vi "T90 Test Konfig.vi"() -> ()   [LabVIEW 2020, in "EPA 1065.lvlib" / "T90 Test 1065-308.lvlib"]
uses:
  T90 Test 1065-308.lvlib
  T90 Konfig Daten.ctl
  Modus.ctl
  Seiten/System Einstellungen V2/Analysatoren.ctl
  Seiten/System Einstellungen V2/Gasflasche Auswahl.ctl
  Seiten/System Einstellungen V2/Konfig Gasflasche.ctl
  Frequenz.ctl
  Visualisierungs Elemente/Zahlen-Ausgabefeld.ctl
  Ergebnis.ctl
  Aktion FGV T90.ctl
  Seiten/FT-IR/FGV FT-IR Gasliste Aktionen.ctl
  Aktion T90 Zustandsautomat.ctl
  Sprachverwaltung/FGV Aktion Tabelle zerlegen.ctl
  Seiten/System Einstellungen V2/Aktion FGV Gasbottledefinition.ctl
  PDF_Interface/PDF Interface Helper/PDFResultPictures.ctl
  Aktion FGV Datenmanagment.ctl
  Allgemeine VIs/Aktion Wertaenderung Gasliste.ctl
  Result Textfile.ctl
  Allgemeine VIs/Aktion Test Status.ctl
  Funktionstasten/Funktionstasten-Aktion.ctl
  Funktionstasten/Zustaende.ctl
  Allgemein/allgemeine Sub-VIs.lvlib
  Seiten/FT-IR/FT-IR.lvlib
  Funktionstasten/Funktionstasten.lvlib
  Linearisierung V2/Protokoll/Protokoll.lvlib
  EPA 1065.lvlib
  Sprachverwaltung/Sprachverwaltung.lvlib
  Seiten/System Einstellungen V2/System Einstellungen V2.lvlib
  PDF_Interface/PDF Interface Helper/PDF Interface Helper.lvlib
  Seiten/Gaszuordnung AO/Gaszuordnung AO.lvlib
panel:
  out "Ergebnis PDF FALSE":T1 caption="Ergebnis 2"
  out "Ergebnis PDF TRUE":T1 caption="Ergebnis 1"
  out "T90 PDF":waveform(sgl)(graph) caption="T90"
  in  "Systemeinstellung":bool caption="Gasliste geändert"
  in  "Gasliste geändert":bool
  in  "Registerkarte":enum32{"Settings", "T90 Test", "Result"}(tab)
  in  "T90 Konfig Daten":T2={"Bearbeiter:"="", "Komponente:"=0, "Gasflaschen Nr.:"="", "Accuracy"=0.0, "Sollwert"=0.0, "Modus"=0, "Abschaltzeit:"=120.0, "Abweichung:"=3.0, "Pfad:"=path "D:/IAG_Data/Log", "Textname:"="", "CG Aufschaltzeit:"=120.0, "Einheit"="", "N2 Aufschaltzeit:"=120.0, "Analysator"="", "Gasflasche"=0, "Konfig Gasflasche"=FALSE, "Frequency:"=5} {"Frequency:" items=["5 Hz"=5, "10 Hz"=10]; "Gasflasche" items=["----"=10000, "IAG O2"=0, "IAG C2H2"=1, "IAG C2H4"=2, "IAG NH3 200"=3, "IAG NH3 2000"=4, "IAG NH3 3000"=5, "IAG CO 5%"=6, "IAG Propane 2%"=7, "IAG NO 1000"=8, "IAG SO2"=9, "IAG C3H6"=10, "IAG CO2"=11, "IAG CO"=12, "IAG N2O"=13, "IAG N2O 100"=14, "IAG NO2 1000"=15, "IAG NO2 100"=16, "IAG CH4"=17, "IAG Propane"=18, "IAG NO 5000"=19, "Hansi"=20, "IAG MG"=21]; "N2 Aufschaltzeit:" min=30.0; "CG Aufschaltzeit:" min=60.0; "Komponente:" items=["NO (3000) LP 191C", "NO2 (150) LP 191C (1of2)", "NO2 (2000) LP 191C (2of2)", "N2O (300) LP 191C (1of2)", "NH3 (300) LP 191C (1of2)", "NH3 (900,3000) LP 191C (2of2)", "HNCO (400) 191C", "H2O% (30) LP 191C", "Formaldehyde (70,500) LP 191C", "CO2 low% (4) LP 191C (2of2)", "CO2% (20) LP 191C (1of2)", "CO (700) LP 191C (1of3)", "CO% (1) LP 191C (2of3)", "Propylene (1000) LP 191C", "Aromatic HC C7 (500) LP 191C", "Ethylene (1000) LP 191C", "CH4 (250) LP 191C (1of2)", "CH4 (5000) LP 191C (2of2)", "Ethane (1000) LP 191C", "Acetylene (1000) LP 191C", "HNO2 (20) 191C", "MeOH (1000) 191C", "CO% (10) LP 191C (3of3)", "Formic Acid (100) 191C", "SO2 (500) LP 191C", "Acetaldehyde (1000) LP 191C", "COS (100) LP 191C", "1,3 butadiene (100) LP 191C", "Oil as Octane (200) LP 191C", "N2O (1000) LP 191C (2of2)", "Propane (200) LP 191C", "NO2 autorange (2000)", "CO autorange (100000)", "CH4 autorange (5000)", "NH3 autorange (3000)", "NOx autorange (3000)", "HCD (10000)", "NMHCD (10000)", "CO2% autorange (20)", "H2Oppm (300000)", "N2O autorange (1000)", "NMNEHCD (3000)", "Temp. Gascell", "Pressure Gascell", "sBeam@2500", "Temp. HL to FT-IR", "Temp. HL Extern SP1", "Outlet Temp FT-IR", "Temp. Cabinet", "Constant 0", "Constant 50", "Constant 100", "AK DUMMY"]; "Abweichung:" min=2.0; "Abschaltzeit:" min=60.0; "Modus" items=["CG zu PNS", "CG zu Entnahmestelle"]}
  in  "Speichern":bool caption="Save"
  out "Komponente":string caption="Komponente:"
  out "Status":string
  out "T90":waveform(sgl)(graph)
  in  "Test Start":bool
  in  "Abbrechen":bool
  out "Istwert":T8 caption="Istwert:" format="%.2f"
  out "Einheit":string
  out "Averaged T10-T90":string caption="gemittelter T10-T90"
  out "Frequenz 2":string
  out "Averaged T90-T10":string caption="gemittelter T90-T10"
  out "Averaged T90-T10 2":string caption="gemittelter T90-T10"
  out "Averaged T10-T90 2":string caption="gemittelter T10-T90"
  out "Ergebnis 4":T1
  out "Ergebnis 3":T1
  out "Ergebnis 2":T1
  out "Ergebnis 1":T1
  out "Ergebnis x5 (T90 T10)":string caption="Mean T10-T90"
  out "Ergebnis x5 (T10 T90)":string caption="Mean T10-T90"
  out "Frequenz 1":string
  out "Tabelle T0-T90":string[][](table) caption="Tabelle"
  in  "Save to file":bool caption="Abbrechen"
  out "T90 Result":waveform(sgl)(graph) caption="T90"
  in  "Print PDF":bool caption="Abbrechen"
  out "Tabelle":string[][](table)
  # "T90 Test EPA §1065.308"
  # "Editor"
  # "Gas bottle number:"
  # "Übersetzungen:\n\nCG priming Time:\nCG Purge Time:"
  # "Path"
  # "Textname:"
  # "Allgemeine Einstellung"
  # "Protokoll Einstellung"
  # "sec."
  # "sec."
  # "%"
  # "%"
  # "sec."
  # "Grenzen"
  # "Ergebnis"
  # "s"
  # ">5"
  # ">5"
  # "<10s"
  # "<10s"
  # "s"
  # "s"
  # "s"
  # "s"
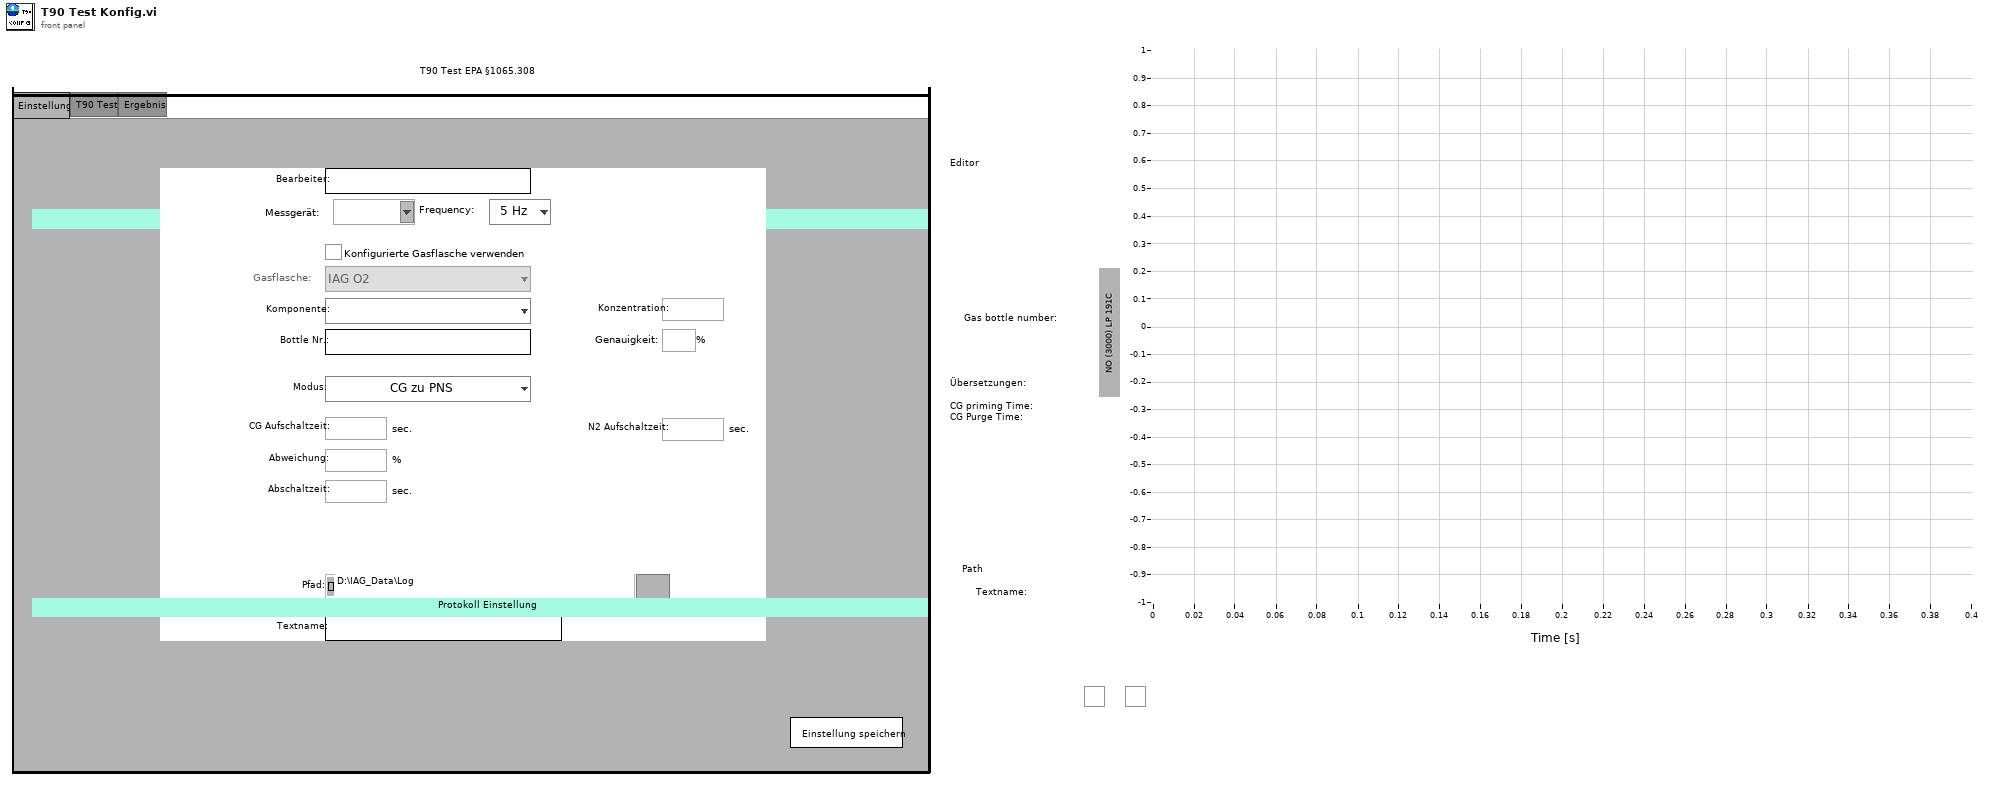
[diagram p1: front panel]
types:
  T1 = typedef "EPA 1065.lvlib/T90 Test 1065-308.lvlib/Ergebnis.ctl" = bool
  T2 = typedef "EPA 1065.lvlib/T90 Test 1065-308.lvlib/T90 Konfig Daten.ctl" = cluster{"Bearbeiter:":string, "Komponente:":u16, "Gasflaschen Nr.:":string, "Accuracy":dbl, "Sollwert":dbl, "Modus":T3, "Abschaltzeit:":dbl, "Abweichung:":dbl, "Pfad:":path, "Textname:":string, "CG Aufschaltzeit:":dbl, "Einheit":string, "N2 Aufschaltzeit:":dbl, "Analysator":T4, "Gasflasche":T5, "Konfig Gasflasche":T6, "Frequency:":T7}
  T3 = typedef "EPA 1065.lvlib/T90 Test 1065-308.lvlib/Modus.ctl" = u16
  T4 = typedef "System Einstellungen V2.lvlib/Analysatoren.ctl" = string
  T5 = typedef "System Einstellungen V2.lvlib/Gasflasche Auswahl.ctl" = u16
  T6 = typedef "System Einstellungen V2.lvlib/Konfig Gasflasche.ctl" = bool
  T7 = typedef "EPA 1065.lvlib/T90 Test 1065-308.lvlib/Frequenz.ctl" = u16
  T8 = typedef "Zahlen-Ausgabefeld.ctl" = sgl
  T9 = typedef "EPA 1065.lvlib/T90 Test 1065-308.lvlib/Aktion FGV T90.ctl" = enum16{"lesen", "Konfig Daten", "speichern", "laden", "T90 aktiv", "T90 inaktiv", "Ext. Ventil aktivieren", "Ext. Ventil deaktivieren", "N2 spülen aktiv", "N2 spülen inaktiv", "Ergebnis Textfile"}
  T10 = typedef "System Einstellungen V2.lvlib/Aktion FGV Gasbottledefinition.ctl" = enum16{"lesen", "schreiben", "löschen", "laden", "speichern", "exportieren", "importieren"}
  T11 = typedef "Sprachverwaltung.lvlib/FGV Aktion Tabelle zerlegen.ctl" = enum16{"laden", "vereinzeln", "speichern"}
  T12 = typedef "EPA 1065.lvlib/T90 Test 1065-308.lvlib/Aktion T90 Zustandsautomat.ctl" = enum16{"init", "start", "CG aufschalten", "Aufschaltzeit einhalten", "Peak ermitteln", "spülen", "CG Sequenz T10", "CG Sequenz T90", "CG halten", "N2 Sequenz T90", "N2 Sequenz T10", "N2 halten", "Auswerten", "abbrechen", "Störung", "fertig"}
  T13 = typedef "FT-IR.lvlib/FGV FT-IR Gasliste Aktionen.ctl" = enum16{"lesen", "Gasliste FT-IR", "Gasliste ausgelesen", "laden", "speichern", "löschen"}
  T14 = typedef "PDF Interface.lvlib/PDF Interface Helper.lvlib/PDFResultPictures.ctl" = cluster{"Yes Ctl Refnum":refnum<vi>, "No Ctl Refnum":refnum<vi>}
  T15 = typedef "String - Ausgabefeld.ctl" = string
  T16 = typedef "System Einstellungen V2.lvlib/Gasflasche gesamt.ctl" = cluster{"Gasflasche":T17, "Trägergas":T18, "Komponenten":T19[]}
  T17 = typedef "System Einstellungen V2.lvlib/Gasflasche.ctl" = cluster{"Gasname für die Auswahl":string, "Chargennummer":string, "Ablaufdatum":timestamp}
  T18 = typedef "System Einstellungen V2.lvlib/Traegergas.ctl" = string
  T19 = typedef "System Einstellungen V2.lvlib/Gasflaschenkomponente.ctl" = cluster{"Gasauswahl":string, "Konzentration IST":dbl, "Einheit":string, "Genauigkeit":dbl}
  T20 = cluster{"Komponente:":u16, "Sollwert":dbl, "Accuracy":dbl, "Einheit":string, "Gasflaschen Nr.:":string}
  T21 = typedef "EPA 1065.lvlib/Aktion Wertaenderung Gasliste.ctl" = enum16{"Init", "lesen", "Gasliste geändert", "ARN inaktiv", "LEAK inaktiv", "Interference 366 inaktiv", "T90 inaktiv", "Interference 375 inaktiv", "Chiller inaktiv", "FID O2 inaktiv", "FID Opti inaktiv", "Drift inaktiv", "Pre Test inaktiv", "LinV2 inaktiv", "HovaCAL Interference inaktiv"}
  T22 = typedef "EPA 1065.lvlib/T90 Test 1065-308.lvlib/Aktion FGV Datenmanagment.ctl" = enum16{"init", "lesen", "Istwerte schreiben", "höchsten Peak setzen", "Auswerten", "Grenzen setzen", "Sollwert ändern", "Rise T10", "Rise T90", "Fall T90", "Fall T10", "Bit löschen", "Umschaltzeitpunkt"}
  T23 = typedef "EPA 1065.lvlib/T90 Test 1065-308.lvlib/Result Textfile.ctl" = cluster{"Averaged T10-T90":string, "Averaged T90-T10":string, "Ergebnis x5 (T10 T90)":string, "Ergebnis x5 (T90 T10)":string, "Ergebnis 1":T1, "Ergebnis 2":T1, "Ergebnis 3":T1, "Ergebnis 4":T1}
  T24 = enum16{"open", "replace", "create", "open or create", "replace or create", "replace or create with confirmation"}
  T25 = typedef "EPA 1065.lvlib/Aktion Test Status.ctl" = enum16{"init", "lesen", "prüfen", "Interference 366", "Interference 375", "Chiller läuft", "Drift läuft", "Pre Test läuft", "FID Optimization läuft", "FID Interference läuft", "HovaCAL Interference", "LinV2"}
  T26 = typedef "Funktionstasten.lvlib/Zustaende.ctl" = enum16{"Standby", "Pause", "Eco", "Messen", "Kalibrieren", "Spülen Filter", "Spülen Leitung", "Umgebungsluft", "0-Gas", "Cal-Gas", "CG zu PNS", "-------------", "Init 1", "Init 2", "Init 3", "Init 4", "Messen vorbereiten", "Messen durchführen", "Exit"}
  T27 = typedef "Funktionstasten.lvlib/Funktionstasten-Aktion.ctl" = enum16{"Initialisieren", "Zustand setzen", "Taste gedrückt", "Fehler speichern", "Lesen", "Manuell", "Remote", "Bitparallel", "Samplepoint", "Zeit Prüfen", "reset Umschalten"}
  T28 = typedef "EPA 1065.lvlib/Aktive Tests Cluster.ctl" = cluster{"ANR läuft":bool, "T90 läuft":bool, "Leak läuft":bool, "Interference 366 läuft":bool, "Interference 375 läuft":bool, "Chiller läuft":bool, "FID Interference läuft":bool, "FID optimization läuft":bool, "Drift läuft":bool, "Pre-test läuft":bool, "HovaCAL Interference läuft":bool, "LinV2 läuft":bool}
  T29 = typedef "EPA 1065.lvlib/T90 Test 1065-308.lvlib/Datencluster.ctl" = cluster{"Höchster Peak":T30, "T10 Grenzwert":T30, "T90 Grenzwert":T30, "Rise Times":dbl[], "Fall Times":dbl[], "RiseTime gemittelt":T30, "FallTime gemittelt":T30, "Zeitstempel":timestamp[], "Rise T10":bool, "Rise T90":bool, "Fall T10":bool, "Fall T90":bool, "RiseTime >5":bool, "Falltime >5":bool, "RiseTime <10":bool, "Falltime <10":bool, "T0-T90":dbl[], "T100-T10":dbl[]}
  T30 = typedef "Zahlen-Eingabefeld.ctl" = sgl
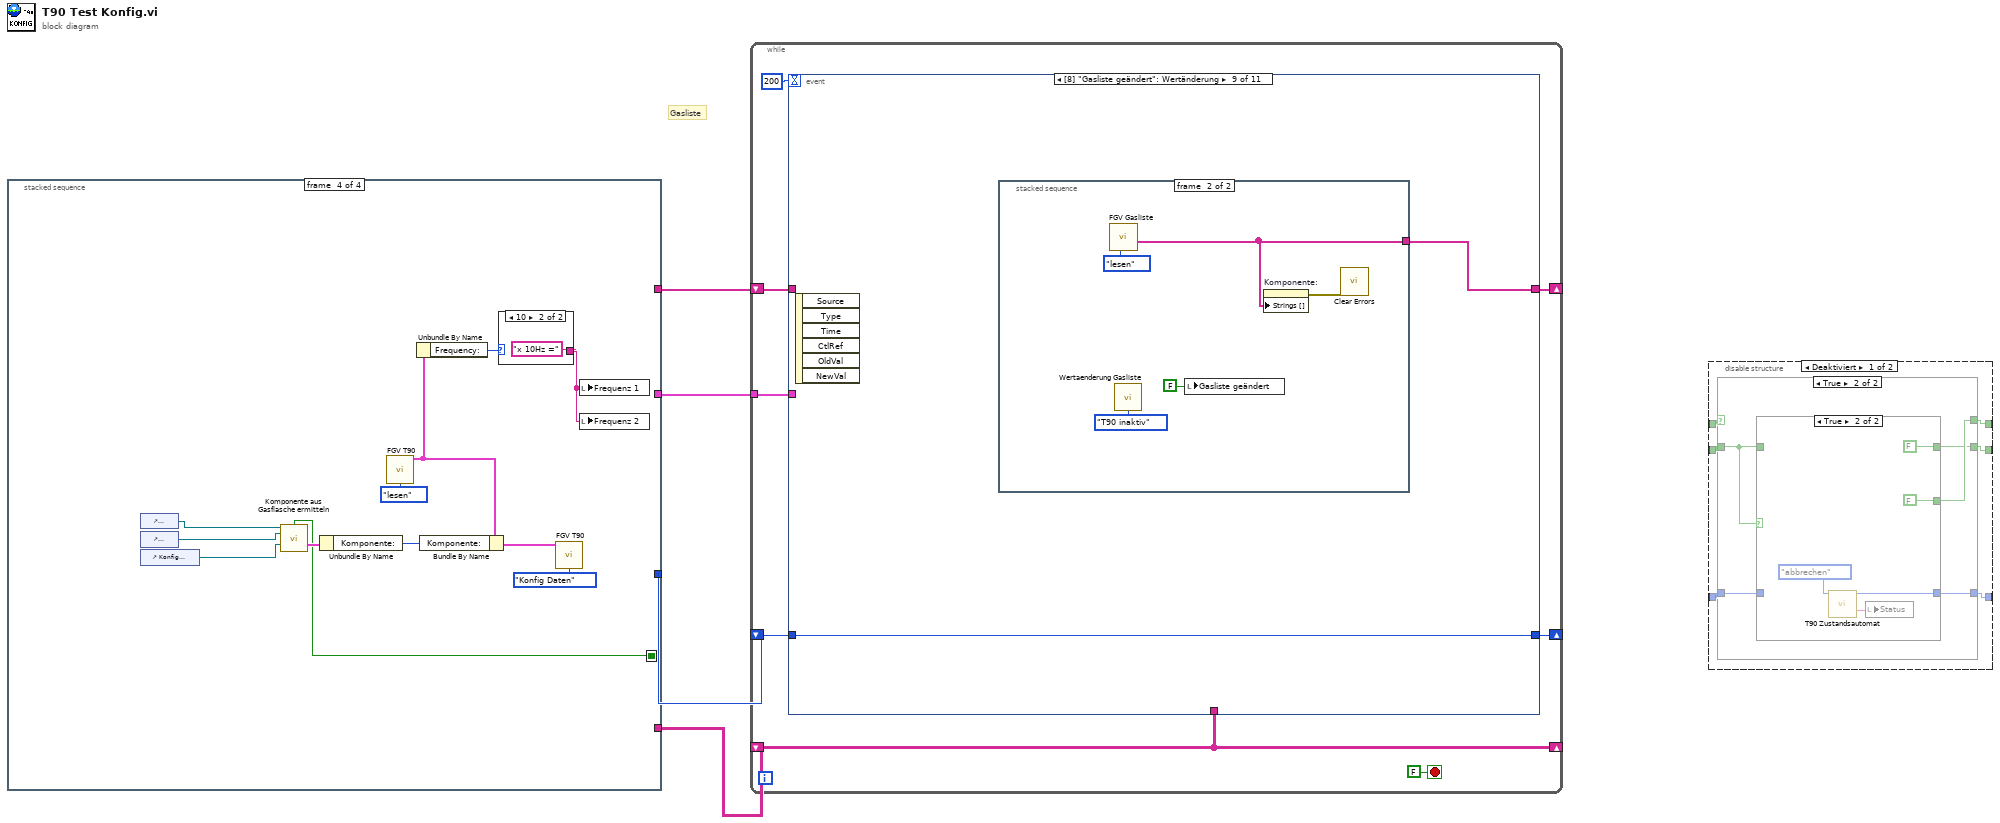
[diagram p0: block diagram]
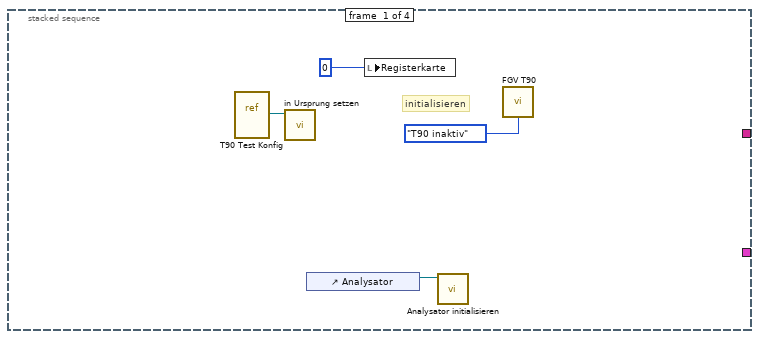
[diagram p2: hidden frame]
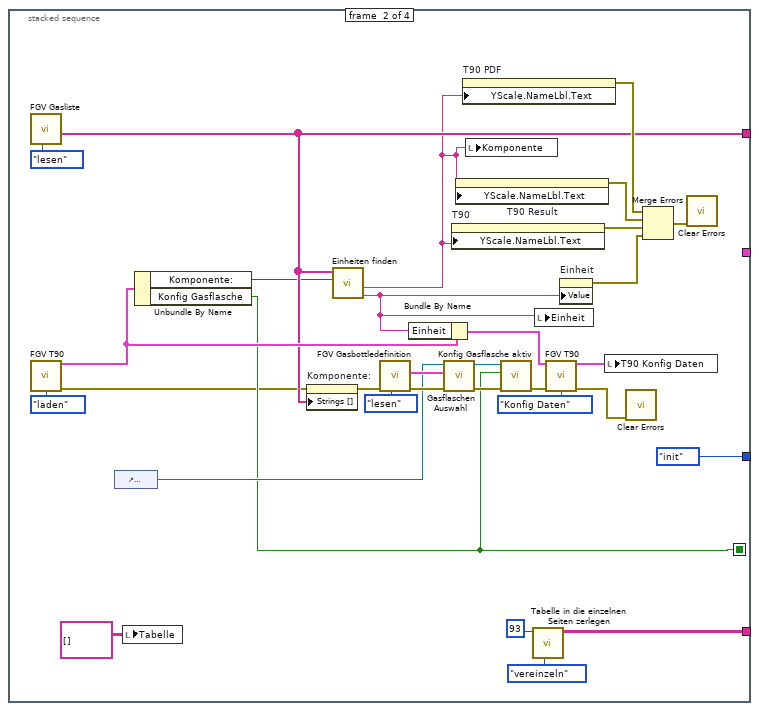
[diagram p3: hidden frame]
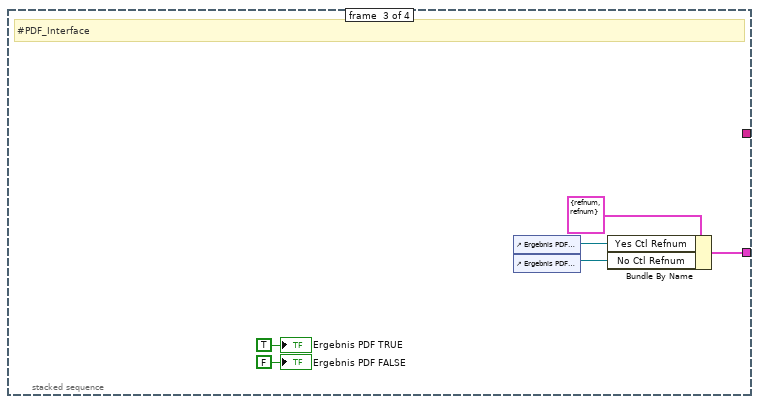
[diagram p4: hidden frame]
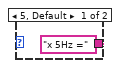
[diagram p5: hidden frame]
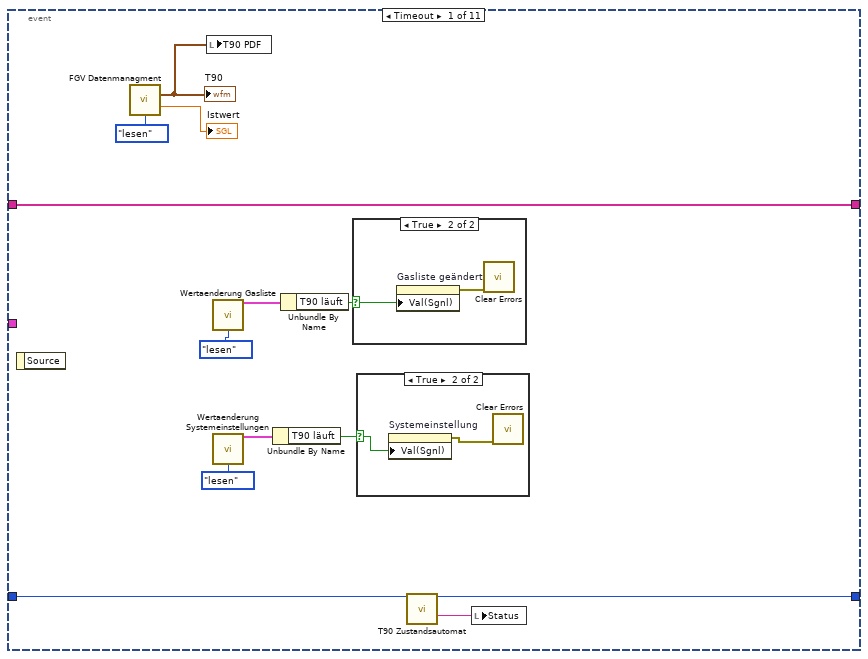
[diagram p6: hidden frame]
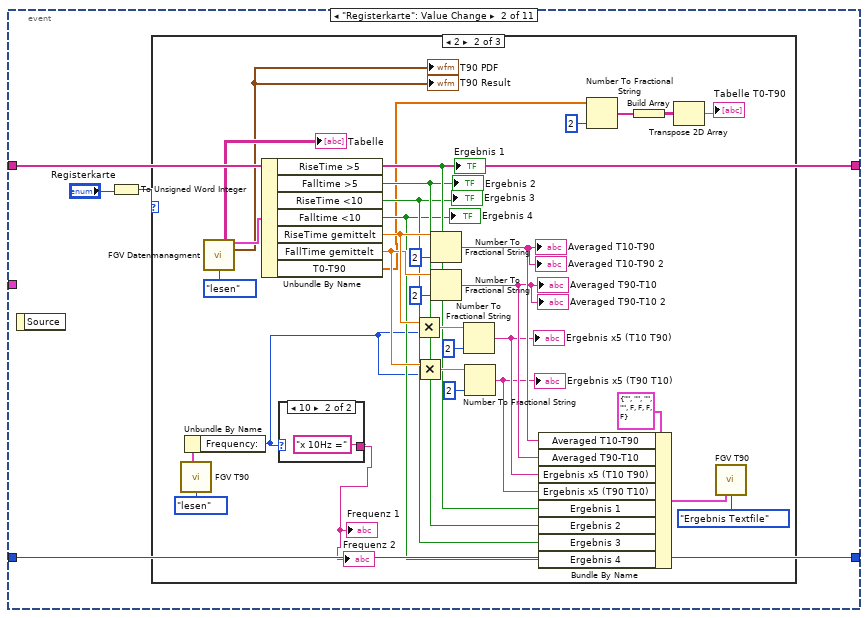
[diagram p9: hidden frame]
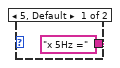
[diagram p11: hidden frame]
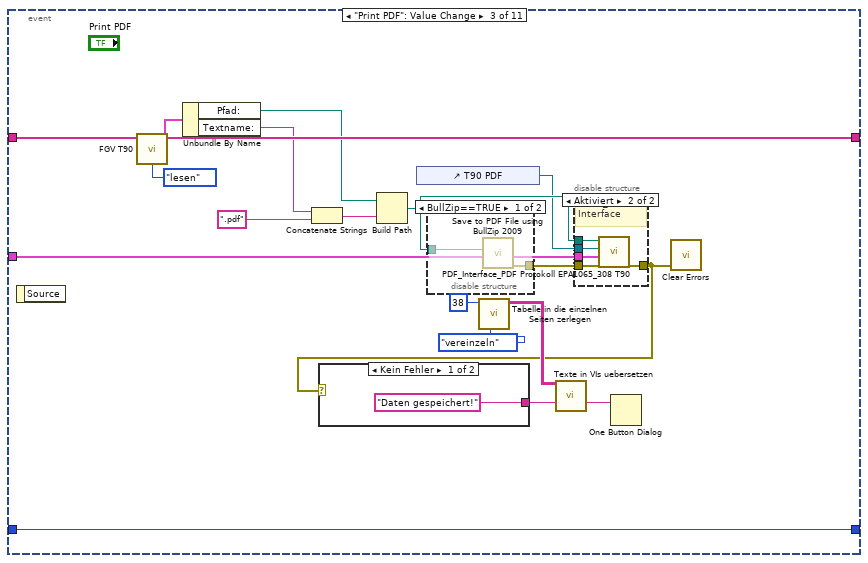
[diagram p13: hidden frame]
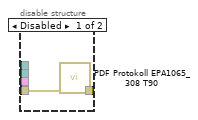
[diagram p14: hidden frame]
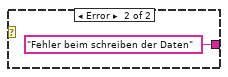
[diagram p15: hidden frame]
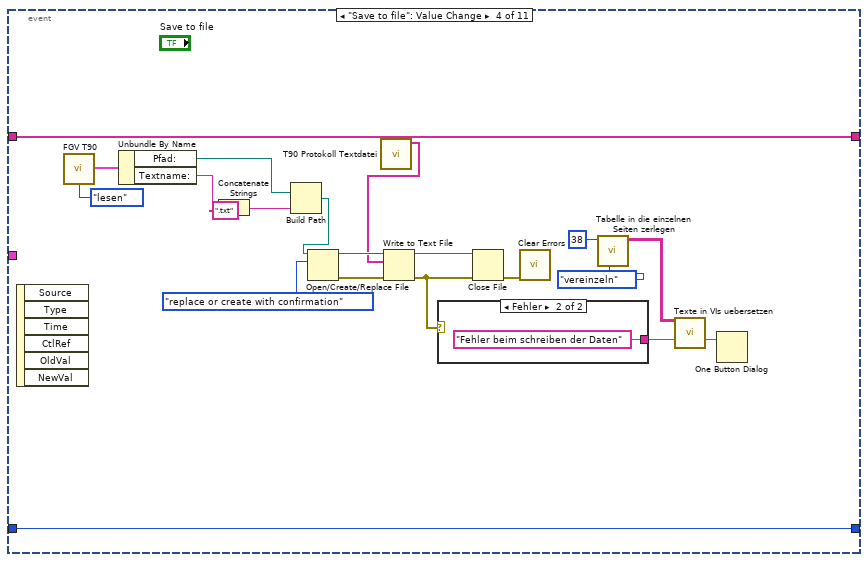
[diagram p17: hidden frame]
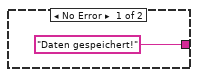
[diagram p18: hidden frame]
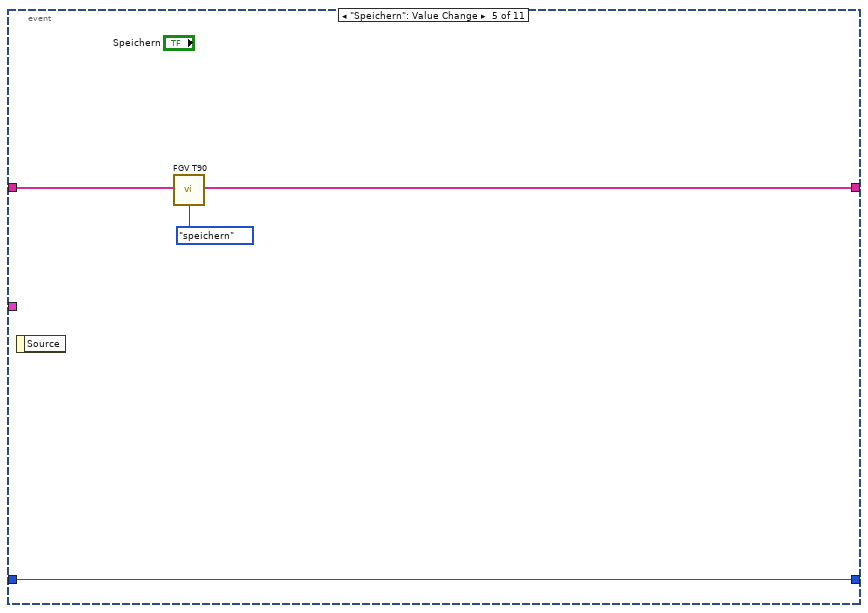
[diagram p19: hidden frame]
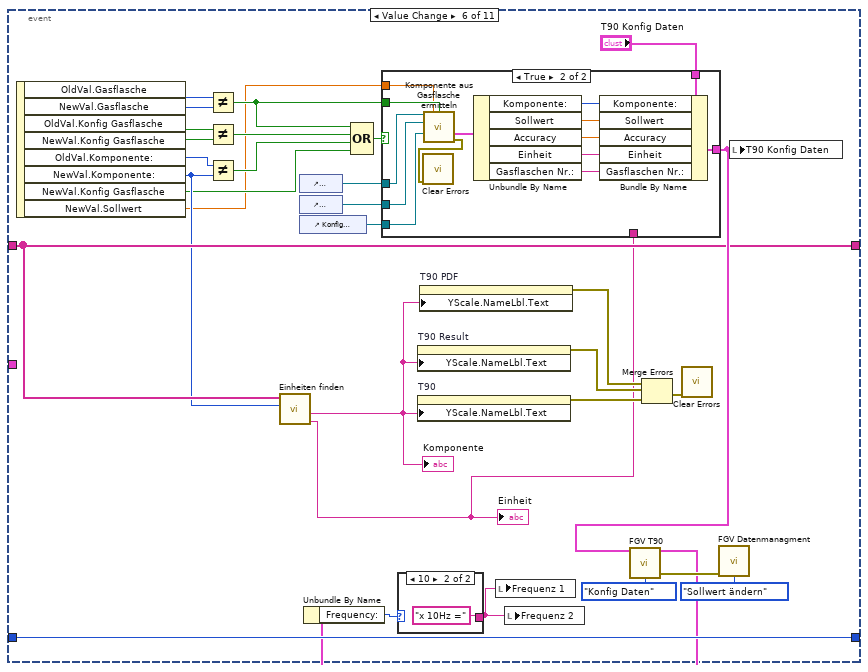
[diagram p20: hidden frame]
diagram:
  # "Gasliste"
  n1 = stacked-sequence {
    seq-local: [_ w16 _ _] -> [_ _ _ w48]
    tunnel: [_ w13 _ _] -> w4
    tunnel: [_ Aktion_T90_Zustandsautomat."init" ("Aktion") _ _] -> w3
    tunnel: [_ w26 _ _] -> w2
    tunnel: [_ _ w39 _] -> w1
    frame #0 {
      # "initialisieren"
      n2 = vi-ref "T90 Test Konfig.vi"() -> (w6:refnum<vi>)
      n3 = call "in Ursprung setzen.vi"("VI Referenz"=w6) -> ()  [unwired: 10 in, 1 out]
      n4 = control-ref of="Analysator"() -> (w5:refnum<vi>)
      n5 = local write "Registerkarte"(0) -> ()
      n6 = call "Analysator initialisieren.vi"("Referenz Analysator"=w5) -> ()  [unwired: 9 in, 2 out]
      n7 = call "FGV T90.vi"("Aktion"=Aktion_FGV_T90."T90 inaktiv") -> ()  [unwired: 9 in, 6 out]
    }
    frame #1 {
      n8 = call "FGV Gasliste.vi"("Aktionen"=FGV_FT-IR_Gasliste_Aktionen."lesen") -> ("Aktuelle Gasliste gesamt"=w13:T15[])  [unwired: 8 in, 2 out]
      n9 = call "FGV T90.vi"("Aktion"=Aktion_FGV_T90."laden") -> ("T90 Konfig Daten"=w25:T2, "error out"=w9:errorcluster)  [unwired: 9 in, 4 out]
      n10 = control-ref of="Gasflasche"() -> (w22:refnum<vi>)
      n11 = local write "Tabelle"(string[][] [] ("Tabellenelement")) -> ()
      n12 = Unbundle By Name(w25) -> ("Komponente:"=w12:u16, "Konfig Gasflasche"=w16:T6)
      n13 = property on="Komponente:" class="Ring (strikt)"(error in=w9, "Strings []"=w13) -> (error out=w17:errorcluster)  [unwired: 1 in, 1 out]
      n14 = call "Einheiten finden.vi"("Komponente"=w12, "Aktuelle Gasliste gesamt"=w13) -> ("Einheit in String"=w10:string, "Komponenten Name"=w11:T15)  [unwired: 8 in]
      n15 = call "FGV Gasbottledefinition.vi"("Aktion"=Aktion_FGV_Gasbottledefinition."lesen", "error in (no error)"=w17) -> ("error out"=w23:errorcluster, "Gasflaschen Liste gesamt"=w24:T16[])  [unwired: 7 in, 1 out]
      n16 = Bundle By Name(cluster=w25, "Einheit"=w10) -> (w30:T2)
      n17 = call "Gasflaschen Auswahl.vi"("error in (no error)"=w23, "Gasflaschen Liste gesamt"=w24, "Ring (Eingang)"=w22) -> ("error out"=w19:errorcluster)  [unwired: 8 in]
      n18 = property on="T90" class="SVGraph (strikt)"("YScale.NameLbl.Text"=w11) -> (error out=w35:errorcluster)  [unwired: 2 in, 1 out]
      n19 = property on="T90 Result" class="SVGraph (strikt)"("YScale.NameLbl.Text"=w11) -> (error out=w33:errorcluster)  [unwired: 2 in, 1 out]
      n20 = property on="T90 PDF" class="SVGraph (strikt)"("YScale.NameLbl.Text"=w11) -> (error out=w14:errorcluster)  [unwired: 2 in, 1 out]
      n21 = local write "Komponente"(w11) -> ()
      n22 = call "Konfig Gasflasche aktiv.vi"("error in (no error)"=w19, "Konfig Gasflasche"=w16, "Referenz Gasflasche"=w22) -> ("error out"=w18:errorcluster)  [unwired: 8 in]
      n23 = call "Tabelle in die einzelnen Seiten zerlegen.vi"("Aktion"=FGV_Aktion_Tabelle_zerlegen."vereinzeln", "Index (Seite)"=93) -> ("Sprachliste"=w26:string[][])  [unwired: 7 in, 2 out]
      n24 = local write "Einheit"(w10) -> ()
      n25 = call "FGV T90.vi"("T90 Konfig Daten"=w30, "error in (no error)"=w18, "Aktion"=Aktion_FGV_T90."Konfig Daten") -> ("T90 Konfig Daten"=w29:T2, "error out"=w20:errorcluster)  [unwired: 7 in, 4 out]
      n26 = property on="Einheit" class="Str"("Value"=w10) -> (error out=w15:errorcluster)  [unwired: 2 in, 1 out]
      n27 = local write "T90 Konfig Daten"(w29) -> ()
      n28 = call <vilib>:"Clear Errors.vi"("error in (no error)"=w20) -> ()  [unwired: 5 in, 2 out]
      n29 = Merge Errors(w14, w33, w35, w15) -> (w34:errorcluster)
      n30 = call <vilib>:"Clear Errors.vi"("error in (no error)"=w34) -> ()  [unwired: 5 in, 2 out]
    }
    frame #2 {
      # "#PDF_Interface"
      n31 = control-ref of="Ergebnis PDF TRUE"() -> (w41:refnum<vi>)
      n32 = control-ref of="Ergebnis PDF FALSE"() -> (w40:refnum<vi>)
      n33 = Bundle By Name(cluster=T14 {"Yes Ctl Refnum"=refnum, "No Ctl Refnum"=refnum} ("ResultPictures"), "Yes Ctl Refnum"=w41, "No Ctl Refnum"=w40) -> (w39:T14)
      "Ergebnis PDF TRUE" <- T1 TRUE ("Ergebnis PDF TRUE")
      "Ergebnis PDF FALSE" <- T1 FALSE ("Ergebnis PDF FALSE")
    }
    frame #3 {
      n34 = control-ref of="Gasflasche"() -> (w51:refnum<vi>)
      n35 = control-ref of="Komponente:"() -> (w50:refnum<vi>)
      n36 = control-ref of="Konfig Gasflasche"() -> (w49:refnum<vi>)
      n37 = call "Komponente aus Gasflasche ermitteln.vi"("Referenz Gasflasche"=w51, "Wertänderung Gasflasche"=w48, "Referenz Komponente"=w50, "Referenz Konfig Gasflasche"=w49) -> ("Ausgangs-Cluster"=w54:T20)  [unwired: 8 in, 3 out]
      n38 = Unbundle By Name(w54) -> ("Komponente:"=w53:u16)
      n39 = call "FGV T90.vi"("Aktion"=Aktion_FGV_T90."lesen") -> ("T90 Konfig Daten"=w46:T2)  [unwired: 9 in, 5 out]
      n40 = Unbundle By Name(w46) -> ("Frequency:"=w47:T7)
      n41 = Bundle By Name(cluster=w46, "Komponente:"=w53) -> (w52:T2)
      n42 = case shown="10" w47 {
        tunnel: ["x 5Hz =" "x 10Hz ="] -> w45
        frame 5, Default {
        }
        frame 10 {
        }
      }
      n43 = call "FGV T90.vi"("T90 Konfig Daten"=w52, "Aktion"=Aktion_FGV_T90."Konfig Daten") -> ()  [unwired: 8 in, 6 out]
      n44 = local write "Frequenz 1"(w45) -> ()
      n45 = local write "Frequenz 2"(w45) -> ()
    }
  }
  n46 = while {
    shift-right: [w63] -> _
    shift-left: w4 -> [w64]
    shift-right: [w61] -> _
    shift-left: w3 -> [w62]
    shift-right: [w60] -> _
    shift-left: w2 -> [w60]
    tunnel: w1 -> [w59]
    stop <- FALSE stop-if-true
    n47 = event shown="[8] \"Gasliste geändert\": Wertänderung" {
      selector: _ -> [_ _ _ _ _ _ _ _ _ _ _]
      dyn-events: _ -> [_ _ _ _ _ _ _ _ _ _ _]
      timeout: 200 -> [_ _ _ _ _ _ _ _ _ _ _]
      tunnel: w64 -> [w79 w87 w139 w171 w175 w182 w232 w234 _ w249 w264]
      tunnel: [w79 w87 w139 w171 w175 w182 w232 w234 w238 w249 w264] -> w63
      tunnel: w62 -> [w78 w84 w131 w170 w174 w202 w231 w233 w239 _ w262]
      tunnel: [w77 w84 w131 w170 w174 w202 w231 w233 w239 w248 w263] -> w61
      tunnel: w60 -> [_ _ _ _ _ _ _ _ _ w245 _]
      tunnel: w59 -> [_ _ w122 _ _ _ _ _ _ _ _]
      event Timeout {
        n48 = event-data() -> ()  [unwired: 1 in, 1 out]
        n49 = call "FGV Datenmanagment.vi"("Aktion"=Aktion_FGV_Datenmanagment."lesen") -> ("T90 Signalverlauf"=w67:waveform(sgl), "Aktueller Wert"=→"Istwert":sgl)  [unwired: 7 in, 6 out]
        "T90" <- w67
        n50 = local write "T90 PDF"(w67) -> ()
        n51 = call "Wertaenderung Gasliste.vi"("Aktion"=Aktion_Wertaenderung_Gasliste."lesen") -> ("Tests"=w72:T28)  [unwired: 13 in, 1 out]
        n52 = call "Wertaenderung Systemeinstellungen.vi"("Aktion"=Aktion_Wertaenderung_Gasliste."lesen") -> ("Tests"=w69:T28)  [unwired: 13 in, 1 out]
        n53 = Unbundle By Name(w69) -> ("T90 läuft"=w68:bool)
        n54 = Unbundle By Name(w72) -> ("T90 läuft"=w71:bool)
        n55 = case shown="True" w71 {
          selector: w71 -> [_ w83]
          frame False {
          }
          frame True {
            n56 = property on="Gasliste geändert" class="Bool. (strikt)"("Val(Sgnl)"=w83) -> (error out=w82:errorcluster)  [unwired: 2 in, 1 out]
            n57 = call <vilib>:"Clear Errors.vi"("error in (no error)"=w82) -> ()  [unwired: 5 in, 2 out]
          }
        }
        n58 = case shown="True" w68 {
          selector: w68 -> [_ w80]
          frame False {
          }
          frame True {
            n59 = property on="Systemeinstellung" class="Bool. (strikt)"("Val(Sgnl)"=w80) -> (error out=w81:errorcluster)  [unwired: 2 in, 1 out]
            n60 = call <vilib>:"Clear Errors.vi"("error in (no error)"=w81) -> ()  [unwired: 5 in, 2 out]
          }
        }
        n61 = call "T90 Zustandsautomat.vi"("Aktion"=w78) -> ("Aktion"=w77:T12, "Status"=w74:string)  [unwired: 11 in, 2 out]
        n62 = local write "Status"(w74) -> ()
      }
      event "Registerkarte": Value Change {
        n63 = event-data() -> ()  [unwired: 1 in, 1 out]
        n64 = To Unsigned Word Integer(number="Registerkarte") -> (unsigned 16bit integer=w85:u16)
        n65 = case shown="2" w85 {
          frame 0, Default {
          }
          frame 2 {
            n66 = call "FGV T90.vi"("Aktion"=Aktion_FGV_T90."lesen") -> ("T90 Konfig Daten"=w91:T2)  [unwired: 9 in, 5 out]
            n67 = Unbundle By Name(w91) -> ("Frequency:"=w90:T7)
            n68 = call "FGV Datenmanagment.vi"("Aktion"=Aktion_FGV_Datenmanagment."lesen") -> ("Ergebnistabelle"=→"Tabelle":string[][], "Daten"=w117:T29, "T90 Signalverlauf"=→"T90 Result" →"T90 PDF":waveform(sgl))  [unwired: 7 in, 5 out]
            n69 = Unbundle By Name(w117) -> ("RiseTime >5"=w101:bool, "Falltime >5"=w100:bool, "RiseTime <10"=w99:bool, "Falltime <10"=w98:bool, "RiseTime gemittelt"=w110:T30, "FallTime gemittelt"=w109:T30, "T0-T90"=w94:dbl[])
            "Ergebnis 1" <- w101
            "Ergebnis 2" <- w100
            "Ergebnis 4" <- w98
            "Ergebnis 3" <- w99
            n70 = case shown="10" w90 {
              tunnel: ["x 5Hz =" "x 10Hz ="] -> w89
              frame 5, Default {
              }
              frame 10 {
              }
            }
            "Frequenz 2" <- w89
            "Frequenz 1" <- w89
            n71 = Multiply(x=w110, y=w90) -> (x*y=w114:T30)
            n72 = Multiply(x=w109, y=w90) -> (x*y=w113:T30)
            n73 = Number To Fractional String(number=w110, precision (6)=i16 2 ("Genauigkeit (6)")) -> (F-format string=w108:string)  [unwired: 2 in]
            "Averaged T10-T90 2" <- w108
            "Averaged T10-T90" <- w108
            n74 = Number To Fractional String(number=w109, precision (6)=i16 2 ("Genauigkeit (6)")) -> (F-format string=w107:string)  [unwired: 2 in]
            "Averaged T90-T10 2" <- w107
            "Averaged T90-T10" <- w107
            n75 = Number To Fractional String(number=w114, precision (6)=i16 2 ("Genauigkeit (6)")) -> (F-format string=w106:string)  [unwired: 2 in]
            "Ergebnis x5 (T10 T90)" <- w106
            n76 = Number To Fractional String(number=w113, precision (6)=i16 2 ("Genauigkeit (6)")) -> (F-format string=w105:string)  [unwired: 2 in]
            "Ergebnis x5 (T90 T10)" <- w105
            n77 = Bundle By Name(cluster=T23 {"Averaged T10-T90"="", "Averaged T90-T10"="", "Ergebnis x5 (T10 T90)"="", "Ergebnis x5 (T90 T10)"="", "Ergebnis 1"=FALSE, "Ergebnis 2"=FALSE, "Ergebnis 3"=FALSE, "Ergebnis 4"=FALSE} ("Result Textfile"), "Averaged T10-T90"=w108, "Averaged T90-T10"=w107, "Ergebnis x5 (T10 T90)"=w106, "Ergebnis x5 (T90 T10)"=w105, "Ergebnis 1"=w101, "Ergebnis 2"=w100, "Ergebnis 3"=w99, "Ergebnis 4"=w98) -> (w102:T23)
            n78 = Number To Fractional String(number=w94, precision (6)=i16 2 ("Genauigkeit (6)")) -> (F-format string=w96:string[])  [unwired: 2 in]
            n79 = Build Array(w96) -> (w95:string[][])
            n80 = Transpose 2D Array(2D array=w95) -> (transposed array=→"Tabelle T0-T90":string[][])
            n81 = call "FGV T90.vi"("Result Textfile"=w102, "Aktion"=Aktion_FGV_T90."Ergebnis Textfile") -> ()  [unwired: 8 in, 6 out]
          }
          frame 1 {
          }
        }
      }
      event "Print PDF": Value Change {
        n82 = event-data() -> ()  [unwired: 1 in, 1 out]
        n83 = call "FGV T90.vi"("Aktion"=Aktion_FGV_T90."lesen") -> ("T90 Konfig Daten"=w135:T2)  [unwired: 9 in, 5 out]
        n84 = Unbundle By Name(w135) -> ("Pfad:"=w133:path, "Textname:"=w134:string)
        n85 = Concatenate Strings(w134, ".pdf") -> (w138:string)
        n86 = Build Path(base path=w133, name or relative path=w138) -> (appended path=w124:path)
        n87 = control-ref of="T90 PDF"() -> (w123:refnum<vi>)
        n88 = disable-structure shown="BullZip==TRUE" {
          disable-tunnel: w124 -> [w150 _]
          disable-tunnel: [w149 _] -> w132
          frame condition #0 {
            n89 = call "Save to PDF File using BullZip 2009.vi"("Save PDF File Path"=w150) -> ("error out"=w149:errorcluster)  [unwired: 10 in]
          }
          frame condition #1 (active) {
          }
        }
        n90 = call "Tabelle in die einzelnen Seiten zerlegen.vi"("Aktion"=FGV_Aktion_Tabelle_zerlegen."vereinzeln", "Index (Seite)"=38) -> ("Sprachliste"=w128:string[][])  [unwired: 7 in, 2 out]
        n91 = disable-structure shown="Aktiviert" {
          disable-tunnel: w132 -> [w141 w146]
          disable-tunnel: [w140 w145] -> w125
          disable-tunnel: w124 -> [_ w144]
          disable-tunnel: w123 -> [_ w143]
          disable-tunnel: w122 -> [_ w142]
          frame Disabled {
            n92 = call "PDF Protokoll EPA1065_308 T90.vi"("error in (no error)"=w141) -> ("error out"=w140:errorcluster)  [unwired: 10 in]
          }
          frame Enabled {
            # "#PDF_Interface"
            n93 = call "PDF_Interface_PDF Protokoll EPA1065_308 T90.vi"("error in (no error)"=w146, "ResultPictures"=w142, "SVGraph Referenz"=w143, "Save PDF File Path"=w144) -> ("error out"=w145:errorcluster)  [unwired: 7 in]
          }
        }
        n94 = case shown="Kein Fehler" w125 {
          tunnel: ["Daten gespeichert!" ("String") "Fehler beim schreiben der Daten" ("String")] -> w129
          frame No Error {
          }
          frame Error {
          }
        }
        n95 = call "Texte in VIs uebersetzen.vi"("Sprachliste"=w128, "String zum Übersetzen"=w129) -> ("String zum Übersetzen"=w130:string)  [unwired: 9 in, 4 out]
        n96 = One Button Dialog(message=w130) -> ()  [unwired: 1 in, 1 out]
        n97 = call <vilib>:"Clear Errors.vi"("error in (no error)"=w125) -> ()  [unwired: 5 in, 2 out]
      }
      event "Save to file": Value Change {
        n98 = event-data() -> ()  [unwired: 1 in, 6 out]
        n99 = call "FGV T90.vi"("Aktion"=Aktion_FGV_T90."lesen") -> ("T90 Konfig Daten"=w166:T2)  [unwired: 9 in, 5 out]
        n100 = Unbundle By Name(w166) -> ("Pfad:"=w164:path, "Textname:"=w165:string)
        n101 = Concatenate Strings(w165, ".txt") -> (w169:string)
        n102 = Build Path(base path=w164, name or relative path=w169) -> (appended path=w152:path)
        n103 = Open/Create/Replace File(file path (use dialog)=w152, operation (0:open)=T24."replace or create with confirmation" ("Operation (0:Öffnen)")) -> (refnum out=w156:refnum<file>, error out=w157:errorcluster)  [unwired: 4 in, 1 out]
        n104 = call "T90 Protokoll Textdatei.vi"() -> ("Textdatei"=w151:string[])  [unwired: 11 in]
        n105 = Write to Text File(file (use dialog)=w156, text=w151, error in=w157) -> (refnum out=w159:refnum<file>, error out=w160:errorcluster)  [unwired: 1 in, 1 out]
        n106 = case shown="Fehler" w160 {
          tunnel: ["Daten gespeichert!" ("String") "Fehler beim schreiben der Daten" ("String")] -> w162
          frame No Error {
          }
          frame Error {
          }
        }
        n107 = Close File(refnum=w159, error in=w160) -> (error out=w158:errorcluster)  [unwired: 1 out]
        n108 = call <vilib>:"Clear Errors.vi"("error in (no error)"=w158) -> ()  [unwired: 5 in, 2 out]
        n109 = call "Tabelle in die einzelnen Seiten zerlegen.vi"("Aktion"=FGV_Aktion_Tabelle_zerlegen."vereinzeln", "Index (Seite)"=38) -> ("Sprachliste"=w161:string[][])  [unwired: 7 in, 2 out]
        n110 = call "Texte in VIs uebersetzen.vi"("Sprachliste"=w161, "String zum Übersetzen"=w162) -> ("String zum Übersetzen"=w163:string)  [unwired: 9 in, 4 out]
        n111 = One Button Dialog(message=w163) -> ()  [unwired: 1 in, 1 out]
      }
      event "Speichern": Value Change {
        n112 = event-data() -> ()  [unwired: 1 in, 1 out]
        n113 = call "FGV T90.vi"("Aktion"=Aktion_FGV_T90."speichern") -> ()  [unwired: 9 in, 6 out]
      }
      event Value Change {
        n114 = event-data() -> ("OldVal.Gasflasche"=w197:T5, "NewVal.Gasflasche"=w196:T5, "OldVal.Konfig Gasflasche"=w200:T6, "NewVal.Konfig Gasflasche"=w199:T6, "OldVal.Komponente:"=w195:u16, "NewVal.Komponente:"=w181:u16, "NewVal.Konfig Gasflasche"=w178:T6, "NewVal.Sollwert"=w177:dbl)  [unwired: 1 in]
        n115 = Not Equal?(x=w197, y=w196) -> (x != y?=w194:bool)
        n116 = Not Equal?(x=w200, y=w199) -> (x != y?=w193:T6)
        n117 = Not Equal?(x=w195, y=w181) -> (x != y?=w192:bool)
        n118 = call "Einheiten finden.vi"("Komponente"=w181, "Aktuelle Gasliste gesamt"=w182) -> ("Einheit in String"=w179:string, "Komponenten Name"=w180:T15)  [unwired: 8 in]
        "Komponente" <- w180
        "Einheit" <- w179
        n119 = control-ref of="Gasflasche"() -> (w187:refnum<vi>)
        n120 = control-ref of="Komponente:"() -> (w188:refnum<vi>)
        n121 = control-ref of="Konfig Gasflasche"() -> (w189:refnum<vi>)
        n122 = Compound Arithmetic op=OR ("Mehrfacharithmetik")(w194, w193, w192, w178) -> (w191:T6)
        n123 = case shown="True" w191 {
          tunnel: "T90 Konfig Daten" -> [w211 w225]
          tunnel: [w210 w224] -> w190
          tunnel: w194 -> [_ w223]
          tunnel: w189 -> [_ w221]
          tunnel: w188 -> [_ w222]
          tunnel: w187 -> [_ w219]
          tunnel: w179 -> [w212 _]
          tunnel: w177 -> [_ w213]
          frame False {
            n124 = Bundle By Name(cluster=w211, "Einheit"=w212) -> (w210:T2)
          }
          frame True {
            n125 = call "Komponente aus Gasflasche ermitteln.vi"("Referenz Gasflasche"=w219, "Konzentration IST"=w213, "Wertänderung Gasflasche"=w223, "Referenz Komponente"=w222, "Referenz Konfig Gasflasche"=w221) -> ("Ausgangs-Cluster"=w226:T20, "error out"=w220:errorcluster)  [unwired: 7 in, 2 out]
            n126 = call <vilib>:"Clear Errors.vi"("error in (no error)"=w220) -> ()  [unwired: 5 in, 2 out]
            n127 = Unbundle By Name(w226) -> ("Komponente:"=w218:u16, "Sollwert"=w217:dbl, "Accuracy"=w216:dbl, "Einheit"=w215:string, "Gasflaschen Nr.:"=w214:string)
            n128 = Bundle By Name(cluster=w225, "Komponente:"=w218, "Sollwert"=w217, "Accuracy"=w216, "Einheit"=w215, "Gasflaschen Nr.:"=w214) -> (w224:T2)
          }
        }
        n129 = property on="T90 Result" class="SVGraph (strikt)"("YScale.NameLbl.Text"=w180) -> (error out=w203:errorcluster)  [unwired: 2 in, 1 out]
        n130 = property on="T90" class="SVGraph (strikt)"("YScale.NameLbl.Text"=w180) -> (error out=w204:errorcluster)  [unwired: 2 in, 1 out]
        n131 = property on="T90 PDF" class="SVGraph (strikt)"("YScale.NameLbl.Text"=w180) -> (error out=w183:errorcluster)  [unwired: 2 in, 1 out]
        n132 = call "FGV T90.vi"("T90 Konfig Daten"=w190, "Aktion"=Aktion_FGV_T90."Konfig Daten") -> ("T90 Konfig Daten"=w184:T2, "error out"=w201:errorcluster)  [unwired: 8 in, 4 out]
        n133 = Unbundle By Name(w184) -> ("Frequency:"=w185:T7)
        n134 = case shown="10" w185 {
          tunnel: ["x 5Hz =" "x 10Hz ="] -> w186
          frame 5, Default {
          }
          frame 10 {
          }
        }
        n135 = local write "Frequenz 1"(w186) -> ()
        n136 = local write "Frequenz 2"(w186) -> ()
        n137 = Merge Errors(w183, w203, w204) -> (w205:errorcluster)
        n138 = call <vilib>:"Clear Errors.vi"("error in (no error)"=w205) -> ()  [unwired: 5 in, 2 out]
        n139 = call "FGV Datenmanagment.vi"("error in (no error)"=w201, "Aktion"=Aktion_FGV_Datenmanagment."Sollwert ändern") -> ()  [unwired: 6 in, 8 out]
        n140 = local write "T90 Konfig Daten"(w190) -> ()
      }
      event Value Change {
        n141 = event-data() -> ()  [unwired: 1 in, 6 out]
        n142 = property on="Konfig Gasflasche" class="Bool. (strikt)"() -> (error out=w230:errorcluster, "Value"=w229:T6)  [unwired: 2 in, 1 out]
        n143 = control-ref of="Gasflasche"() -> (w228:refnum<vi>)
        n144 = call "Konfig Gasflasche aktiv.vi"("error in (no error)"=w230, "Konfig Gasflasche"=w229, "Referenz Gasflasche"=w228) -> ("error out"=w227:errorcluster)  [unwired: 8 in]
        n145 = call <vilib>:"Clear Errors.vi"("error in (no error)"=w227) -> ()  [unwired: 5 in, 2 out]
      }
      event "Systemeinstellung": Value Change {
        n146 = event-data() -> ()  [unwired: 1 in, 6 out]
        n147 = stacked-sequence {
          frame #0 {
          }
          frame #1 {
            n148 = control-ref of="Analysator"() -> (w235:refnum<vi>)
            n149 = call "Analysator initialisieren.vi"("Referenz Analysator"=w235) -> ()  [unwired: 9 in, 2 out]
          }
          frame #2 {
            n150 = call "Wertaenderung Systemeinstellungen.vi"("Aktion"=Aktion_Wertaenderung_Gasliste."T90 inaktiv") -> ()  [unwired: 13 in, 2 out]
            n151 = local write "Systemeinstellung"(FALSE ("Systemeinstellung")) -> ()
          }
        }
      }
      event "Gasliste geändert": Value Change {
        n152 = event-data() -> ()  [unwired: 1 in, 6 out]
        n153 = stacked-sequence {
          tunnel: [_ w242] -> w238
          frame #0 {
          }
          frame #1 {
            n154 = call "FGV Gasliste.vi"("Aktionen"=FGV_FT-IR_Gasliste_Aktionen."lesen") -> ("Aktuelle Gasliste gesamt"=w242:T15[])  [unwired: 8 in, 2 out]
            n155 = call "Wertaenderung Gasliste.vi"("Aktion"=Aktion_Wertaenderung_Gasliste."T90 inaktiv") -> ()  [unwired: 13 in, 2 out]
            n156 = local write "Gasliste geändert"(FALSE ("Gasliste geändert")) -> ()
            n157 = property on="Komponente:" class="Ring (strikt)"("Strings []"=w242) -> (error out=w243:errorcluster)  [unwired: 2 in, 1 out]
            n158 = call <vilib>:"Clear Errors.vi"("error in (no error)"=w243) -> ()  [unwired: 5 in, 2 out]
          }
        }
      }
      event "Test Start": Value Change {
        n159 = event-data() -> ()  [unwired: 1 in, 1 out]
        n160 = call "Test Status.vi"("Aktion"=Aktion_Test_Status."lesen") -> ("Tests sperren"=w246:bool)  [unwired: 11 in, 3 out]
        n161 = case shown="False" w246 {
          tunnel: [Aktion_T90_Zustandsautomat."start" ("Aktion") Aktion_T90_Zustandsautomat."init" ("Aktion")] -> w248
          tunnel: w245 -> [_ w252]
          frame False {
            n162 = invoke on="Status" class="Str" method="Std wiederherstellen"() -> (error out=w250:errorcluster)  [unwired: 3 in, 2 out]
            n163 = call <vilib>:"Clear Errors.vi"("error in (no error)"=w250) -> ()  [unwired: 5 in, 2 out]
          }
          frame True {
            n164 = call "Texte in VIs uebersetzen.vi"("Sprachliste"=w252, "String zum Übersetzen"="Anderer Test läuft gerade.\nBitte etwas Geduld." ("Nachricht")) -> ("String zum Übersetzen"=w253:string)  [unwired: 9 in, 4 out]
            n165 = One Button Dialog(message=w253, button name ("OK")="OK" ("Schaltflächentext (\"OK\")")) -> ()  [unwired: 1 out]
          }
        }
      }
      event "Abbrechen": Value Change {
        n166 = event-data() -> ()  [unwired: 1 in, 1 out]
        n167 = call "Test Status.vi"("Aktion"=Aktion_Test_Status."lesen") -> ("Aktive Tests"=w260:T28, "Tests sperren"=w258:bool)  [unwired: 11 in, 2 out]
        n168 = Unbundle By Name(w260) -> ("T90 läuft"=w259:bool)
        n169 = And(x=w259, y=w258) -> (x .and. y?=w257:bool)
        n170 = case shown="False" w257 {
          tunnel: [w265 Aktion_T90_Zustandsautomat."abbrechen" ("Aktion")] -> w263
          tunnel: w262 -> [w265 _]
          frame False {
          }
          frame True {
            n171 = call "FGV-Funktionstasten.vi"("Herkunft"="T90", "Zustand"=Zustaende."Standby", "Aktion"=Funktionstasten-Aktion."Zustand setzen") -> ()  [unwired: 5 in, 8 out]
          }
        }
      }
    }
  }
  n172 = disable-structure shown="Deaktiviert" {
    disable-tunnel: _ -> [w275 _]
    disable-tunnel: [w274 _] -> _
    disable-tunnel: _ -> [w273 _]
    disable-tunnel: [w272 _] -> _
    disable-tunnel: _ -> [w271 _]
    disable-tunnel: [w270 _] -> _
    frame Disabled {
      n173 = case shown="True" w273 {
        selector: w273 -> [w277 _]
        tunnel: w275 -> [_ w283]
        tunnel: [Aktion_T90_Zustandsautomat."init" ("Aktion") w282] -> w274
        tunnel: [w277 w281] -> w272
        tunnel: w271 -> [w276 w280]
        tunnel: [w276 w279] -> w270
        frame False {
        }
        frame True {
          n174 = case shown="True" w280 {
            tunnel: w283 -> [w289 _]
            tunnel: [w288 w294] -> w282
            tunnel: [w286 FALSE] -> w281
            tunnel: [FALSE ("Test Start") FALSE ("Test Start")] -> w279
            tunnel: w280 -> [_ _]
            frame False {
              n175 = call "T90 Zustandsautomat.vi"("Aktion"=w289) -> ("Aktion"=w288:T12, "Status"=→"Status":string)  [unwired: 11 in, 2 out]
              n176 = Not Equal?(x=Aktion_T90_Zustandsautomat."fertig", y=w288) -> (x != y?=w286:bool)
            }
            frame True {
              n177 = call "T90 Zustandsautomat.vi"("Aktion"=Aktion_T90_Zustandsautomat."abbrechen") -> ("Aktion"=w294:T12, "Status"=w293:string)  [unwired: 11 in, 2 out]
              n178 = local write "Status"(w293) -> ()
            }
          }
        }
      }
    }
    frame Enabled {
    }
  }
